vi "Limit Fail.vi"(7 "Channel (1)":i32=1, 8 "error in (no error)":errorcluster, 11 "VISA resource name":refnum<visa-resource-name>) -> (0 "error out":errorcluster, 2 "Limit Fail":bool, 3 "VISA resource name out":refnum<visa-resource-name>)   [LabVIEW 2011, in "Agilent ENA Series.lvlib"]
doc: "Queries a channel limit tests and returns true if the test is failed for the specified channel."
uses:
  Agilent ENA Series.lvlib
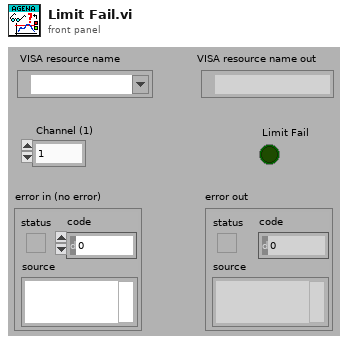
[diagram p1: front panel]
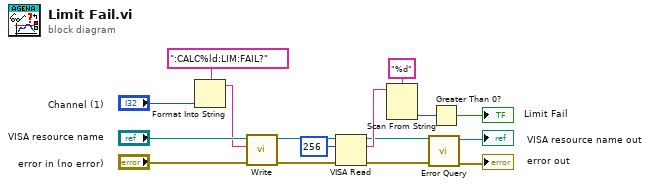
[diagram p0: block diagram]
diagram:
  n1 = Format Into String(format string=":CALC%ld:LIM:FAIL?", "Channel (1)") -> (resulting string=w5:string)  [unwired: 2 in, 1 out]
  n2 = call "Write.vi"("error in (no error)"="error in (no error)", "String ()"=w5, "VISA resource name"="VISA resource name") -> ("error out"=w13:errorcluster, "VISA resource name out"=w14:refnum<visa-resource-name>)  [unwired: 6 in, 1 out]
  n3 = VISA Read(VISA resource name=w14, byte count=u32 256, error in (no error)=w13) -> (VISA resource name out=w4:refnum<visa-resource-name>, read buffer=w11:string, error out=w3:errorcluster)  [unwired: 1 out]
  n4 = Scan From String(format string="%d", input string=w11) -> (output 1=w9:i32)  [unwired: 3 in, 3 out]
  n5 = call "Error Query.vi"("error in (no error)"=w3, "VISA resource name"=w4) -> ("error out"=→"error out":errorcluster, "VISA resource name out"=→"VISA resource name out":refnum<visa-resource-name>)  [unwired: 6 in, 2 out]
  n6 = Greater Than 0?(x=w9) -> (x > 0?=→"Limit Fail":bool)
